vi "tokenize string.vi"(10 "delimiter":string="/", 11 "raw path":string) -> (3 "segments":string[](array[string]))   [LabVIEW 2013, in "uniform resource locator.lvlib"]
uses:
  uniform resource locator.lvlib
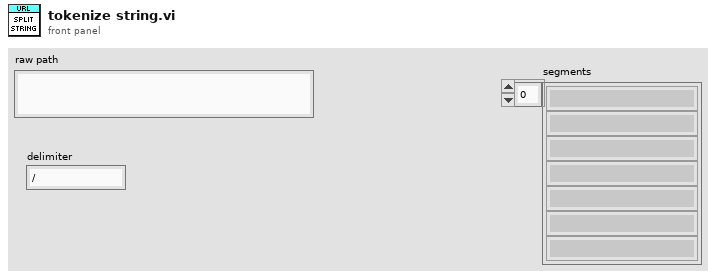
[diagram p1: front panel]
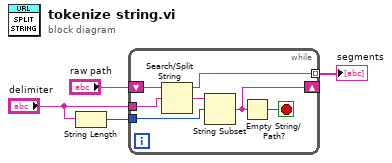
[diagram p0: block diagram]
diagram:
  n1 = String Length(string="delimiter") -> (length=w1:i32)
  n2 = while {
    shift-right: [w8] -> _
    shift-left: "raw path" -> [w11]
    tunnel: [w9] -> w3 mode=indexing
    tunnel: "delimiter" -> [w6]
    tunnel: w1 -> [w5]
    stop <- w7 stop-if-true
    n3 = Search/Split String(string=w11, search string/char (-)=w6) -> (substring before match=w9:string, match + rest of string=w10:string)  [unwired: 1 in, 1 out]
    n4 = String Subset(string=w10, offset (0)=w5) -> (substring=w8:string)  [unwired: 1 in]
    n5 = Empty String/Path?(string/path=w8) -> (empty?=w7:bool)
  }
  "segments" <- w3
